vi "Set Blob Metadata.vi"(6 "Blob Metadata":T1[](array[typedef]), 8 "error in (no error)":errorcluster, 9 "Blob":string, 10 "Container":string, 11 "Azure Session in":refnum<class "Session.lvclass">) -> (0 "error out":errorcluster, 3 "Azure Session out":refnum<class "Session.lvclass">)   [LabVIEW 2015, in "NI_Azure_Blob.lvlib"]
doc: "Sets user-defined metadata of an existing blob."
uses:
  NI_Azure_Blob.lvlib
  Core/Session/Session.lvclass
  Core/Name Value Pair.ctl
  Core/Session/Session.lvclass/Session.ctl
  Core/Session/Write Request Headers.vi
  Core/Session/Write Request Parameters.vi
  Core/Session/Write HTTP Verb.vi
  Core/Session/Write URL Suffix.vi
  Core/NI_Azure_Core.lvlib
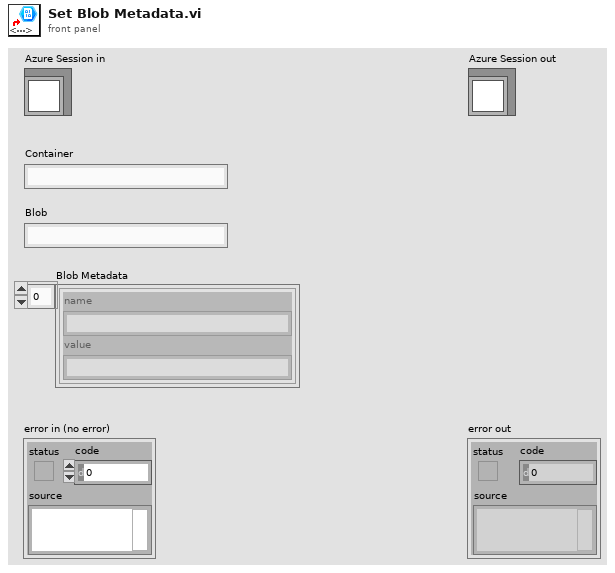
[diagram p1: front panel]
types:
  T1 = typedef "NI_Azure_Core.lvlib/Name Value Pair.ctl" = cluster{"name":string, "value":string}
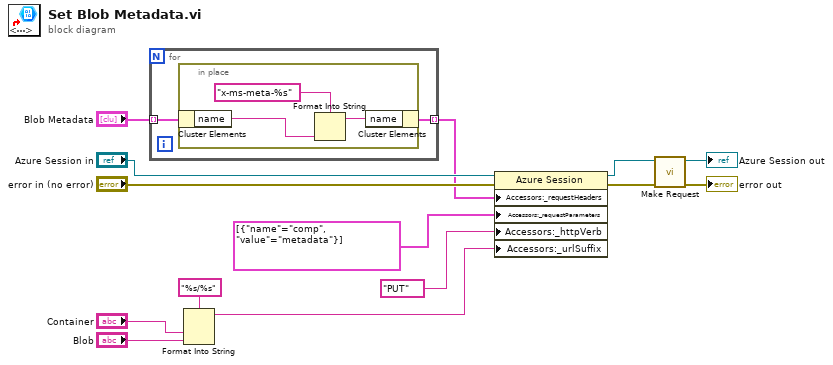
[diagram p0: block diagram]
diagram:
  n1 = for {
    tunnel: "Blob Metadata" -> [w16] mode=indexing
    tunnel: [w15] -> w3 mode=indexing
    n2 = in-place {
      n3 = in-place-cluster #1(w16) -> ("name"=w18:string)
      n4 = Format Into String(format string="x-ms-meta-%s" ("name"), w18) -> (resulting string=w17:string)  [unwired: 2 in, 1 out]
      n5 = in-place-cluster #1("name"=w17) -> (w15:T1)
    }
  }
  n6 = Format Into String(format string="%s/%s", "Container", "Blob") -> (resulting string=w1:string)  [unwired: 2 in, 1 out]
  n7 = property class="Azure Session"(reference="Azure Session in", error in="error in (no error)", "Accessors:_requestHeaders"=w3, "Accessors:_requestParameters"=T1[] [{"name"="comp", "value"="metadata"}] ("request parameters"), "Accessors:_httpVerb"="PUT" ("HTTP-Verb"), "Accessors:_urlSuffix"=w1) -> (reference out=w5:refnum<class "Session.lvclass">, error out=w7:errorcluster)
  n8 = call "Make Request.vi"("error in (no error)"=w7, "Session in"=w5) -> ("error out"=→"error out":errorcluster, "Session out"=→"Azure Session out":refnum<class "Session.lvclass">)  [unwired: 7 in, 1 out]
